vi "T_per_min2A_per_S.vi"(1 "T/min":dbl format="%.4f") -> (0 "A/sec":dbl format="%.1f")   [LabVIEW 2020]
uses:
  PS Comm Globals.vi
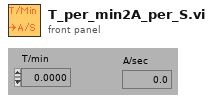
[diagram p1: front panel]
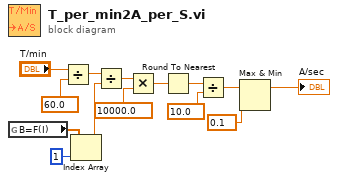
[diagram p0: block diagram]
diagram:
  n1 = global read "PS Comm Globals.vi" "B=F(I)"() -> (w4:dbl[])
  n2 = Divide(x="T/min", y=60.0 ("x")) -> (x/y=w2:dbl)
  n3 = Index Array(array=w4, index=1 ("Index")) -> (element=w1:dbl)
  n4 = Divide(x=w2, y=w1) -> (x/y=w3:dbl)
  n5 = Multiply(x=w3, y=10000.0) -> (x*y=w11:dbl)
  n6 = Round To Nearest(number=w11) -> (nearest integer value=w10:dbl)
  n7 = Divide(x=w10, y=10.0) -> (x/y=w8:dbl)
  n8 = Max & Min(x=w8, y=0.1) -> (max(x,y)=→"A/sec":dbl)  [unwired: 1 out]
